vi "Cursor Control.vi"(7 "플랫폼 조합키":T1, 8 "참조":refnum<vi>, 9 "Num Pad":bool, 10 "ScanCode":i16, 11 "error in":errorcluster caption="error out") -> (0 "참조 출력":refnum<vi>, 3 "error out":errorcluster)   [LabVIEW 2020]
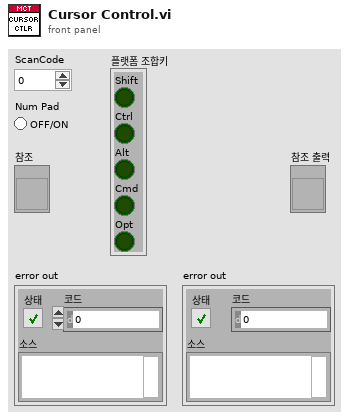
[diagram p1: front panel]
types:
  T1 = cluster{"Shift":bool, "Ctrl":bool, "Alt":bool, "Cmd":bool, "Opt":bool}
  T2 = typedef "LVRowAndColumnTypeDef.ctl" = cluster{"Row":i32, "Column":i32}
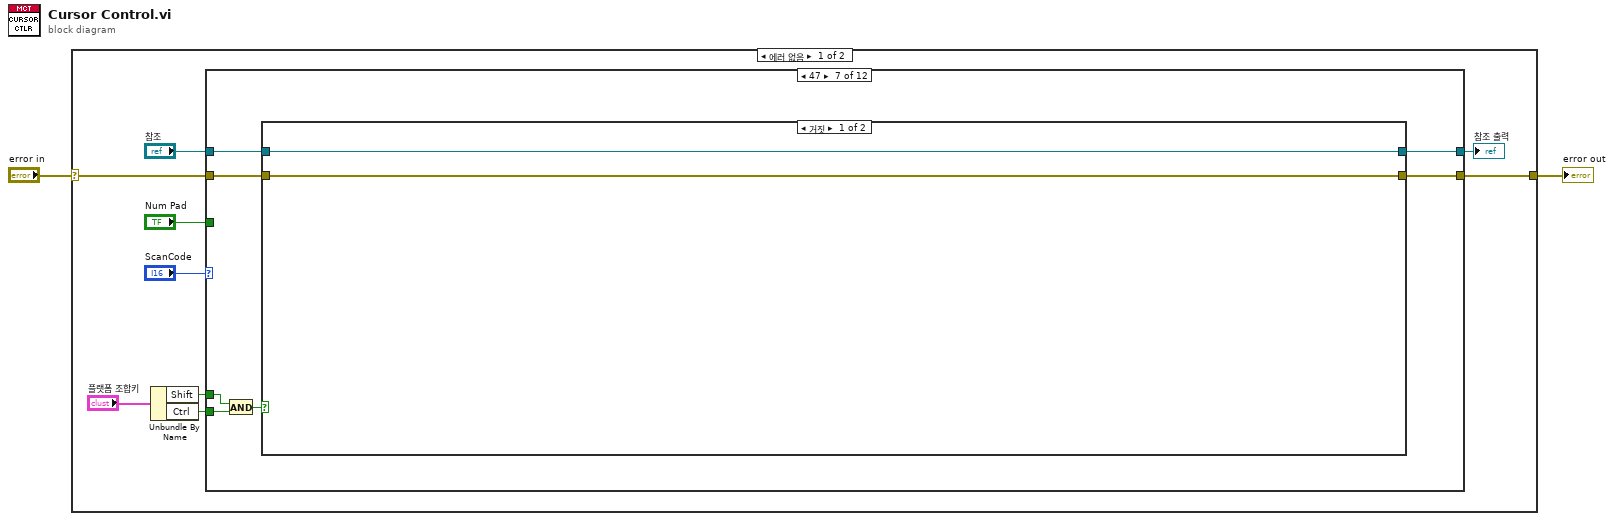
[diagram p0: block diagram]
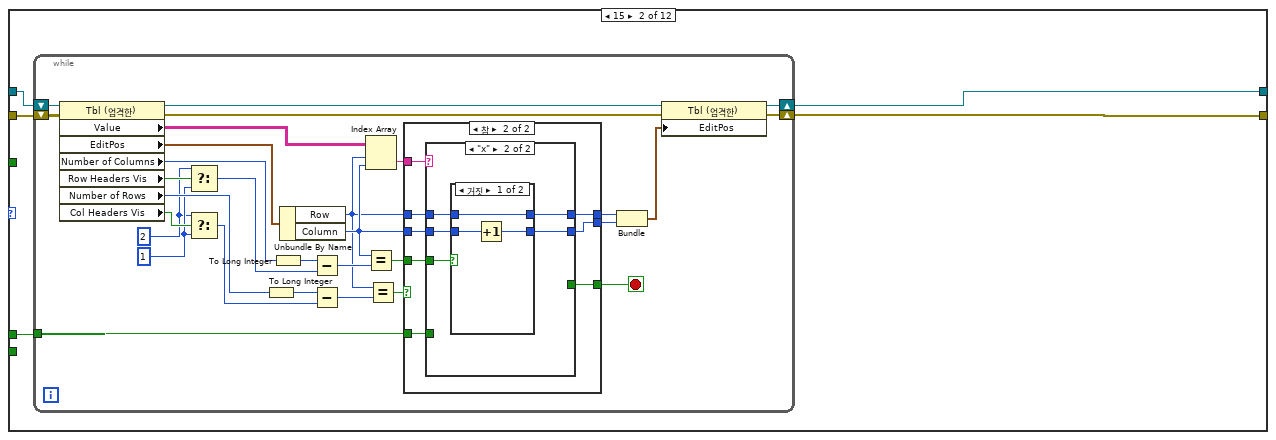
[diagram p3: hidden frame]
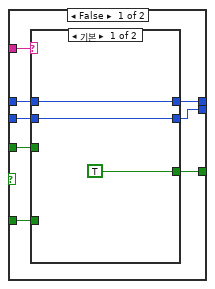
[diagram p4: hidden frame]
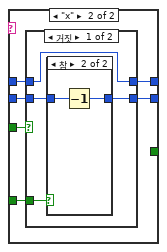
[diagram p5: hidden frame]
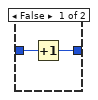
[diagram p6: hidden frame]
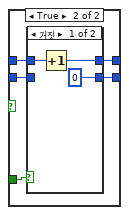
[diagram p7: hidden frame]
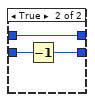
[diagram p8: hidden frame]
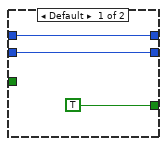
[diagram p9: hidden frame]
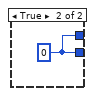
[diagram p10: hidden frame]
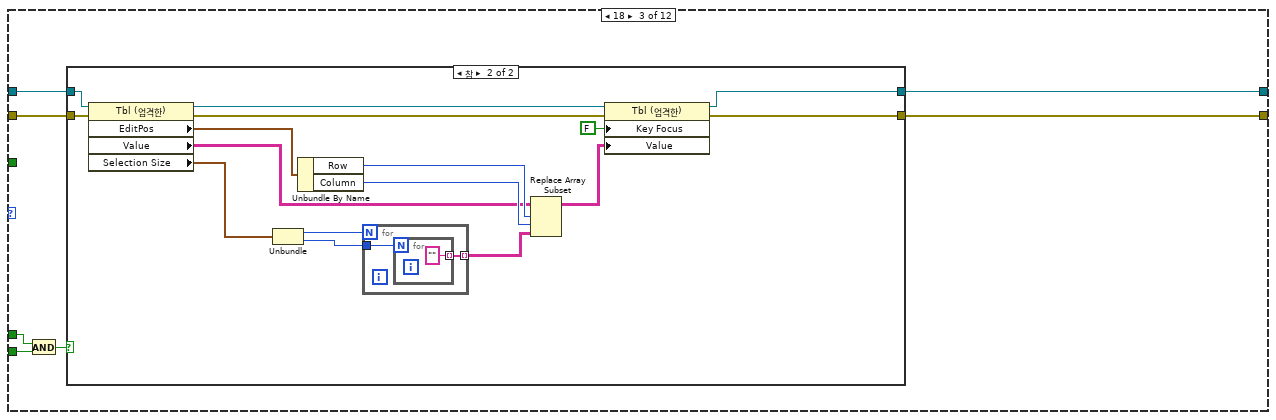
[diagram p11: hidden frame]
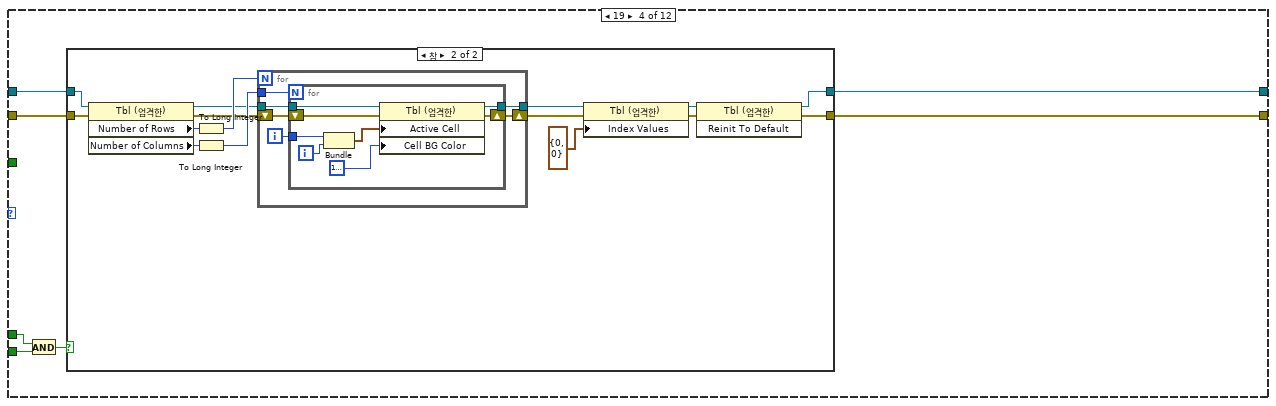
[diagram p13: hidden frame]
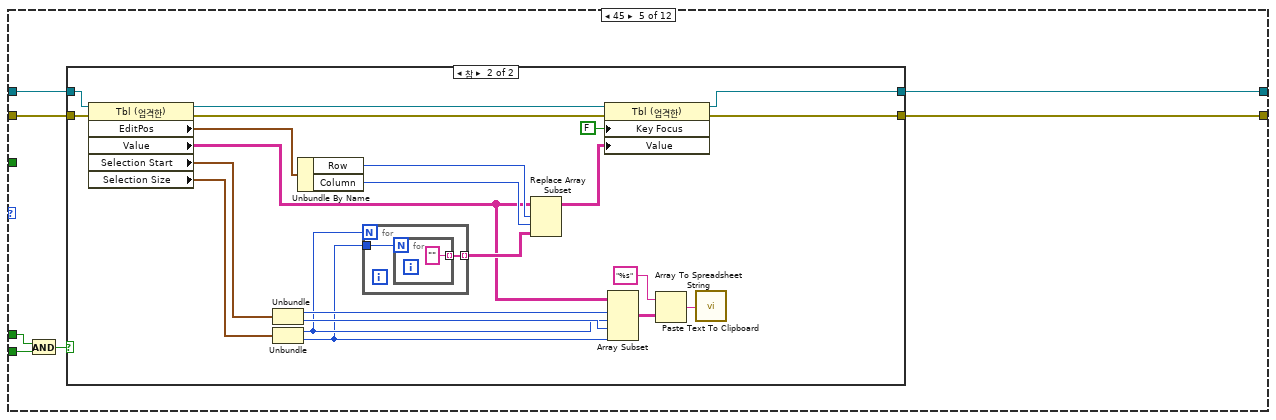
[diagram p15: hidden frame]
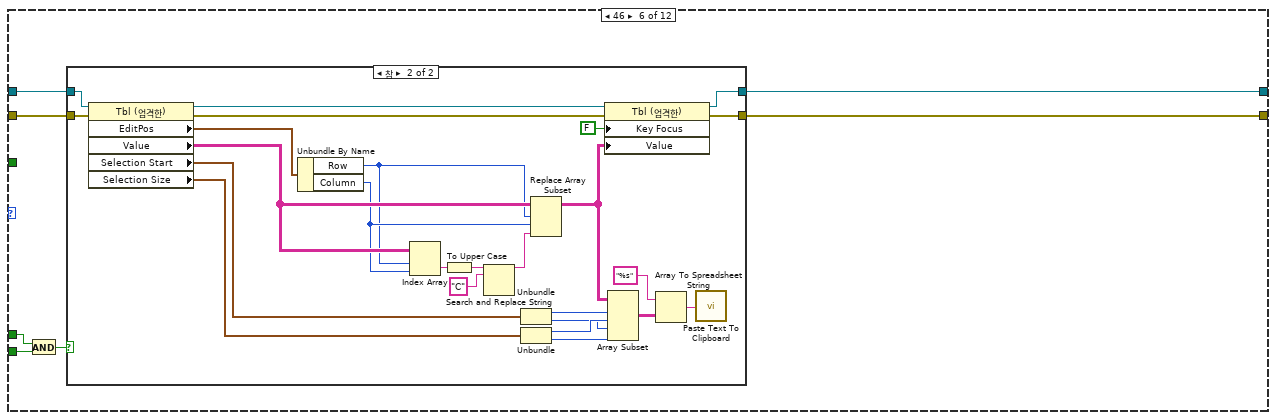
[diagram p17: hidden frame]
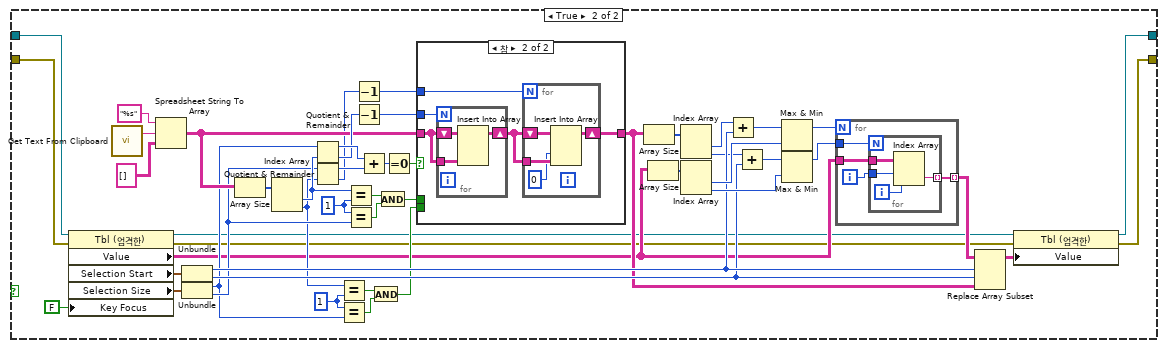
[diagram p19: hidden frame]
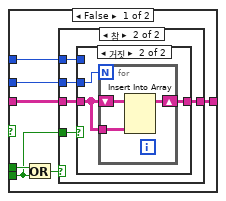
[diagram p20: hidden frame]
diagram:
  n1 = case shown="에러 없음" "error in" {
    selector: "error in" -> [w6 w515]
    tunnel: [w11 w515] -> w2
    frame No Error {
      n2 = Unbundle By Name("플랫폼 조합키") -> ("Shift"=w4:bool, "Ctrl"=w3:bool)
      n3 = case shown="47" "ScanCode" {
        tunnel: w6 -> [w13 w18 w108 w136 w174 w208 w242 w347 w365 w383 w412 w494]
        tunnel: [w13 w16 w106 w134 w172 w206 w240 w346 w364 w382 w411 w493] -> w11
        tunnel: "Num Pad" -> [_ _ _ _ _ _ _ w345 w363 w381 w410 w492]
        tunnel: "참조" -> [w12 w17 w107 w135 w173 w207 w241 w343 w362 w380 w409 w491]
        tunnel: [w12 w15 w105 w133 w171 w205 w239 w344 w361 w379 w408 w490] -> w8
        tunnel: w4 -> [_ w14 w110 w138 w176 w210 w244 _ _ _ w407 _]
        tunnel: w3 -> [_ _ w109 w137 w175 w209 w243 _ _ _ _ _]
        frame Default {
        }
        frame 15 {
          n4 = while {
            shift-right: [w43] -> w16
            shift-left: w18 -> [w47]
            shift-right: [w41] -> w15
            shift-left: w17 -> [w46]
            tunnel: w14 -> [w25]
            stop <- w37 stop-if-true
            w21 = 2 ("y")
            w22 = 1 ("y")
            n5 = property class="Tbl (엄격한)"(reference=w46, error in=w47) -> (reference out=w42:refnum<vi>, error out=w43:errorcluster, "Value"=w45:string[][], "EditPos"=w36:T2, "Number of Columns"=w35:u32, "Row Headers Vis"=w24:bool, "Number of Rows"=w30:u32, "Col Headers Vis"=w23:bool)
            n6 = Select(t=w21, s=w24, f=w22) -> (s? t:f=w20:i32)
            n7 = Select(t=w21, s=w23, f=w22) -> (s? t:f=w19:i32)
            n8 = To Long Integer(number=w30) -> (32bit integer=w26:i32)
            n9 = To Long Integer(number=w35) -> (32bit integer=w28:i32)
            n10 = Unbundle By Name(w36) -> ("Row"=w31:i32, "Column"=w34:i32)
            n11 = Subtract(x=w28, y=w20) -> (x-y=w33:i32)
            n12 = Subtract(x=w26, y=w19) -> (x-y=w29:i32)
            n13 = Index Array(array=w45, index (row)=w31, index (col)=w34) -> (element=w44:string)
            n14 = Equal?(x=w34, y=w33) -> (x = y?=w32:bool)
            n15 = Equal?(x=w31, y=w29) -> (x = y?=w27:bool)
            n16 = case shown="참" w27 {
              tunnel: w44 -> [w55 w91]
              tunnel: [w54 w88] -> w40
              tunnel: [w53 w87] -> w39
              tunnel: [w52 w86] -> w37
              tunnel: w34 -> [w51 w89]
              tunnel: w32 -> [w50 w85]
              tunnel: w31 -> [w49 w90]
              tunnel: w25 -> [w48 w84]
              frame False {
                n17 = case shown="기본" w55 {
                  tunnel: w49 -> [w58 w61]
                  tunnel: w51 -> [w57 w64]
                  tunnel: [w58 w60] -> w54
                  tunnel: [w57 w63] -> w53
                  tunnel: [TRUE _] -> w52
                  tunnel: w50 -> [_ w62]
                  tunnel: w48 -> [_ w59]
                  frame Default {
                  }
                  frame "ⅹ" {
                    n18 = case shown="거짓" w62 {
                      tunnel: w64 -> [w68 w73]
                      tunnel: [w67 w74] -> w63
                      tunnel: w61 -> [w66 w77]
                      tunnel: [w66 w76] -> w60
                      tunnel: w59 -> [w65 w75]
                      frame False {
                        n19 = case shown="참" w65 {
                          tunnel: w68 -> [w70 w72]
                          tunnel: [w69 w71] -> w67
                          frame False {
                            n20 = Increment(x=w70) -> (x+1=w69:i32)
                          }
                          frame True {
                            n21 = Decrement(x=w72) -> (x-1=w71:i32)
                          }
                        }
                      }
                      frame True {
                        n22 = case shown="거짓" w75 {
                          tunnel: w77 -> [w80 w83]
                          tunnel: [w79 w83] -> w76
                          tunnel: [0 w81] -> w74
                          tunnel: w73 -> [_ w82]
                          frame False {
                            n23 = Increment(x=w80) -> (x+1=w79:i32)
                          }
                          frame True {
                            n24 = Decrement(x=w82) -> (x-1=w81:i32)
                          }
                        }
                      }
                    }
                  }
                }
              }
              frame True {
                n25 = case shown="\"ⅹ\"" w91 {
                  tunnel: w90 -> [w94 w96]
                  tunnel: w89 -> [w93 w99]
                  tunnel: [w94 w95] -> w88
                  tunnel: [w93 w98] -> w87
                  tunnel: [TRUE _] -> w86
                  tunnel: w85 -> [_ w97]
                  tunnel: w84 -> [_ _]
                  frame Default {
                  }
                  frame "ⅹ" {
                    n26 = case shown="거짓" w97 {
                      tunnel: w99 -> [w102 _]
                      tunnel: [w101 w103] -> w98
                      tunnel: w96 -> [w100 _]
                      tunnel: [w100 w103] -> w95
                      frame False {
                        n27 = Increment(x=w102) -> (x+1=w101:i32)
                      }
                      frame True {
                        w103 = 0
                      }
                    }
                  }
                }
              }
            }
            n28 = Bundle("Row"=w40, "Column"=w39) -> (w38:cluster{"Row":i32, "Column":i32})  [unwired: 1 in]
            n29 = property class="Tbl (엄격한)"(reference=w42, error in=w43, "EditPos"=w38) -> (reference out=w41:refnum<vi>)  [unwired: 1 out]
          }
        }
        frame 18 {
          n30 = And(x=w110, y=w109) -> (x .and. y?=w104:bool)
          n31 = case shown="참" w104 {
            tunnel: w108 -> [w112 w125]
            tunnel: w107 -> [w111 w126]
            tunnel: [w112 w127] -> w106
            tunnel: [w111 w128] -> w105
            frame False {
            }
            frame True {
              n32 = property class="Tbl (엄격한)"(reference=w126, error in=w125) -> (reference out=w120:refnum<vi>, error out=w121:errorcluster, "EditPos"=w122:T2, "Value"=w113:string[][], "Selection Size"=w117:T2)
              n33 = Unbundle(w117) -> ("Row"=w116:i32, "Column"=w115:i32)
              n34 = Unbundle By Name(w122) -> ("Row"=w123:i32, "Column"=w124:i32)
              n35 = for {
                N: w116 -> [_]
                tunnel: w115 -> [w130]
                tunnel: [w129] -> w114 mode=indexing
                n36 = for {
                  N: w130 -> [_]
                  tunnel: [""] -> w129 mode=indexing
                }
              }
              n37 = Replace Array Subset(array=w113, new element=w114, index (row)=w123, index (col)=w124) -> (w118:string[][])
              n38 = property on="프로퍼티 노드" class="Tbl (엄격한)"(reference=w120, error in=w121, "Key Focus"=FALSE ("키 포커스"), "Value"=w118) -> (reference out=w128:refnum<vi>, error out=w127:errorcluster)
            }
          }
        }
        frame 19 {
          n39 = And(x=w138, y=w137) -> (x .and. y?=w132:bool)
          n40 = case shown="참" w132 {
            tunnel: w136 -> [w140 w149]
            tunnel: w135 -> [w139 w150]
            tunnel: [w140 w141] -> w134
            tunnel: [w139 w142] -> w133
            frame False {
            }
            frame True {
              n41 = property class="Tbl (엄격한)"(reference=w150, error in=w149) -> (reference out=w145:refnum<vi>, error out=w146:errorcluster, "Number of Rows"=w148:u32, "Number of Columns"=w147:u32)
              n42 = To Long Integer(number=w148) -> (32bit integer=w151:i32)
              n43 = To Long Integer(number=w147) -> (32bit integer=w152:i32)
              n44 = for {
                N: w151 -> [_]
                tunnel: w145 -> [w160]
                shift-right: [w159] -> w153
                shift-left: w146 -> [w161]
                tunnel: w152 -> [w157]
                tunnel: [w156] -> w154
                i -> [w158]
                n45 = for {
                  N: w157 -> [_]
                  tunnel: w160 -> [w168]
                  shift-right: [w167] -> w159
                  shift-left: w161 -> [w169]
                  tunnel: w158 -> [w165]
                  tunnel: [w162] -> w156
                  i -> [w164]
                  n46 = Bundle(w165, w164) -> (w166:cluster{i32, i32})  [unwired: 1 in]
                  n47 = property class="Tbl (엄격한)"(reference=w168, error in=w169, "Active Cell"=w166, "Cell BG Color"=u32 16777226) -> (reference out=w162:refnum<vi>, error out=w167:errorcluster)
                }
              }
              n48 = property class="Tbl (엄격한)"(reference=w154, error in=w153, "Index Values"=cluster{i32, i32} {0, 0}) -> (reference out=w144:refnum<vi>, error out=w143:errorcluster)
              n49 = invoke class="Tbl (엄격한)" method="Reinit To Default"(reference=w144, error in=w143) -> (reference out=w142:refnum<vi>, error out=w141:errorcluster)  [unwired: 1 in, 1 out]
            }
          }
        }
        frame 45 {
          n50 = And(x=w176, y=w175) -> (x .and. y?=w170:bool)
          n51 = case shown="참" w170 {
            tunnel: w174 -> [w178 w197]
            tunnel: w173 -> [w177 w198]
            tunnel: [w178 w199] -> w172
            tunnel: [w177 w200] -> w171
            frame False {
            }
            frame True {
              n52 = property class="Tbl (엄격한)"(reference=w198, error in=w197) -> (reference out=w186:refnum<vi>, error out=w187:errorcluster, "EditPos"=w188:T2, "Value"=w179:string[][], "Selection Start"=w191:T2, "Selection Size"=w183:T2)
              n53 = Unbundle(w191) -> ("Row"=w192:i32, "Column"=w193:i32)
              n54 = Unbundle(w183) -> ("Row"=w182:i32, "Column"=w181:i32)
              n55 = Unbundle By Name(w188) -> ("Row"=w189:i32, "Column"=w190:i32)
              n56 = for {
                N: w182 -> [_]
                tunnel: w181 -> [w202]
                tunnel: [w201] -> w180 mode=indexing
                n57 = for {
                  N: w202 -> [_]
                  tunnel: [""] -> w201 mode=indexing
                }
              }
              n58 = Replace Array Subset(array=w179, new element=w180, index (row)=w189, index (col)=w190) -> (w184:string[][])
              n59 = property on="프로퍼티 노드" class="Tbl (엄격한)"(reference=w186, error in=w187, "Key Focus"=FALSE ("키 포커스"), "Value"=w184) -> (reference out=w200:refnum<vi>, error out=w199:errorcluster)
              n60 = Array Subset(array=w179, index (row)=w192, length (row)=w182, index (col)=w193, length (col)=w181) -> (w194:string[][])
              n61 = Array To Spreadsheet String(array=w194, 3:"%s" ("format string")) -> (spreadsheet string=w196:string)  [unwired: 1 in]
              n62 = call "Paste Text To Clipboard.vi"("Text to copy to clipboard"=w196) -> ()  [unwired: 1 out]
            }
          }
        }
        frame 46 {
          n63 = And(x=w210, y=w209) -> (x .and. y?=w204:bool)
          n64 = case shown="참" w204 {
            tunnel: w208 -> [w212 w234]
            tunnel: w207 -> [w211 w235]
            tunnel: [w212 w236] -> w206
            tunnel: [w211 w237] -> w205
            frame False {
            }
            frame True {
              n65 = property class="Tbl (엄격한)"(reference=w235, error in=w234) -> (reference out=w215:refnum<vi>, error out=w216:errorcluster, "EditPos"=w217:T2, "Value"=w233:string[][], "Selection Start"=w225:T2, "Selection Size"=w224:T2)
              n66 = Unbundle By Name(w217) -> ("Row"=w218:i32, "Column"=w220:i32)
              n67 = Index Array(array=w233, index (row)=w218, index (col)=w220) -> (element=w223:string)
              n68 = To Upper Case(1:w223) -> (0:w222:string)
              n69 = Search and Replace String(input string=w222, search string="C" ("검색 문자열")) -> (result string=w219:string)  [unwired: 6 in, 3 out]
              n70 = Unbundle(w225) -> ("Row"=w226:i32, "Column"=w227:i32)
              n71 = Unbundle(w224) -> ("Row"=w232:i32, "Column"=w228:i32)
              n72 = Replace Array Subset(array=w233, new element=w219, index (row)=w218, index (col)=w220) -> (w214:string[][])
              n73 = property on="프로퍼티 노드" class="Tbl (엄격한)"(reference=w215, error in=w216, "Key Focus"=FALSE ("키 포커스"), "Value"=w214) -> (reference out=w237:refnum<vi>, error out=w236:errorcluster)
              n74 = Array Subset(array=w214, index (row)=w226, length (row)=w232, index (col)=w227, length (col)=w228) -> (w229:string[][])
              n75 = Array To Spreadsheet String(array=w229, 3:"%s" ("format string")) -> (spreadsheet string=w231:string)  [unwired: 1 in]
              n76 = call "Paste Text To Clipboard.vi"("Text to copy to clipboard"=w231) -> ()  [unwired: 1 out]
            }
          }
        }
        frame 47 {
          n77 = And(x=w244, y=w243) -> (x .and. y?=w238:bool)
          n78 = case shown="거짓" w238 {
            tunnel: w242 -> [w246 w254]
            tunnel: w241 -> [w245 w253]
            tunnel: [w246 w256] -> w240
            tunnel: [w245 w255] -> w239
            frame False {
            }
            frame True {
              w260 = 1 ("y")
              w268 = 1 ("y")
              n79 = property class="Tbl (엄격한)"(reference=w253, error in=w254, "Key Focus"=FALSE ("키 포커스")) -> (reference out=w247:refnum<vi>, error out=w248:errorcluster, "Value"=w252:string[][], "Selection Start"=w251:T2, "Selection Size"=w250:T2)
              n80 = call "Get Text From Clipboard.vi"() -> ("Text From Clipboard"=w295:string)  [unwired: 1 out]
              n81 = Spreadsheet String To Array(format string="%s", spreadsheet string=w295, array type (2D Dbl)=string[][] []) -> (array=w280:string[][])  [unwired: 1 in]
              n82 = Unbundle(w251) -> ("Row"=w286:i32, "Column"=w285:i32)
              n83 = Unbundle(w250) -> ("Row"=w258:i32, "Column"=w264:i32)
              n84 = Array Size(array=w280) -> (size(s)=w293:i32[])
              n85 = Index Array(array=w293) -> (element #1=w265:i32, element #2=w259:i32)  [unwired: 2 in]
              n86 = Quotient & Remainder(x=w258, y=w265) -> (x-y*floor(x/y)=w284:i32, floor(x/y)=w281:i32)
              n87 = Quotient & Remainder(x=w264, y=w259) -> (x-y*floor(x/y)=w283:i32, floor(x/y)=w273:i32)
              n88 = Equal?(x=w259, y=w260) -> (x = y?=w261:bool)
              n89 = Equal?(x=w260, y=w258) -> (x = y?=w262:bool)
              n90 = Equal?(x=w265, y=w268) -> (x = y?=w267:bool)
              n91 = Equal?(x=w268, y=w264) -> (x = y?=w266:bool)
              n92 = Decrement(x=w273) -> (x-1=w272:i32)
              n93 = Decrement(x=w281) -> (x-1=w274:i32)
              n94 = Add(x=w284, y=w283) -> (x+y=w282:i32)
              n95 = And(x=w261, y=w262) -> (x .and. y?=w257:bool)
              n96 = And(x=w267, y=w266) -> (x .and. y?=w263:bool)
              n97 = Equal To 0?(x=w282) -> (x = 0?=w279:bool)
              n98 = case shown="참" w279 {
                tunnel: w274 -> [w309 w335]
                tunnel: w280 -> [w311 w334]
                tunnel: [w308 w333] -> w277
                tunnel: w272 -> [w310 w331]
                tunnel: w263 -> [w307 _]
                tunnel: w257 -> [w306 _]
                frame False {
                  n99 = Or(x=w307, y=w306) -> (x .or. y?=w305:bool)
                  n100 = case shown="참" w305 {
                    tunnel: w311 -> [w312 w317]
                    tunnel: w306 -> [_ w316]
                    tunnel: w310 -> [_ w315]
                    tunnel: w309 -> [_ w314]
                    tunnel: [w312 w313] -> w308
                    frame False {
                    }
                    frame True {
                      n101 = case shown="거짓" w316 {
                        tunnel: w317 -> [w320 w327]
                        tunnel: w315 -> [w319 _]
                        tunnel: w314 -> [_ w325]
                        tunnel: [w318 w326] -> w313
                        frame True {
                          n102 = for {
                            N: w319 -> [_]
                            shift-right: [w323] -> w318
                            shift-left: w320 -> [w324]
                            tunnel: w320 -> [w322]
                            n103 = Insert Into Array(array=w324, index (col)=0 ("비활성화된 인덱스 (열)"), new element=w322) -> (w323:string[][])  [unwired: 1 in]
                          }
                        }
                        frame False {
                          n104 = for {
                            N: w325 -> [_]
                            shift-right: [w329] -> w326
                            shift-left: w327 -> [w330]
                            tunnel: w327 -> [w328]
                            n105 = Insert Into Array(array=w330, new element=w328) -> (w329:string[][])  [unwired: 2 in]
                          }
                        }
                      }
                    }
                  }
                }
                frame True {
                  n106 = for {
                    N: w335 -> [_]
                    shift-right: [w340] -> w332
                    shift-left: w334 -> [w342]
                    tunnel: w334 -> [w341]
                    n107 = Insert Into Array(array=w342, new element=w341) -> (w340:string[][])  [unwired: 2 in]
                  }
                  n108 = for {
                    N: w331 -> [_]
                    shift-right: [w337] -> w333
                    shift-left: w332 -> [w339]
                    tunnel: w332 -> [w338]
                    n109 = Insert Into Array(array=w339, index (col)=0 ("비활성화된 인덱스 (열)"), new element=w338) -> (w337:string[][])  [unwired: 1 in]
                  }
                }
              }
              n110 = Array Size(array=w277) -> (size(s)=w278:i32[])
              n111 = Array Size(array=w252) -> (size(s)=w292:i32[])
              n112 = Index Array(array=w278) -> (element #1=w276:i32, element #2=w275:i32)  [unwired: 2 in]
              n113 = Index Array(array=w292) -> (element #1=w288:i32, element #2=w287:i32)  [unwired: 2 in]
              n114 = Add(x=w276, y=w286) -> (x+y=w290:i32)
              n115 = Add(x=w275, y=w285) -> (x+y=w289:i32)
              n116 = Max & Min(x=w290, y=w288) -> (max(x,y)=w271:i32)  [unwired: 1 out]
              n117 = Max & Min(x=w289, y=w287) -> (max(x,y)=w270:i32)  [unwired: 1 out]
              n118 = for {
                N: w271 -> [_]
                tunnel: [w300] -> w269 mode=indexing
                tunnel: w270 -> [w298]
                tunnel: w252 -> [w297]
                i -> [w299]
                n119 = for {
                  N: w298 -> [_]
                  tunnel: [w302] -> w300 mode=indexing
                  tunnel: w299 -> [w304]
                  tunnel: w297 -> [w301]
                  i -> [w303]
                  n120 = Index Array(array=w301, index (row)=w304, index (col)=w303) -> (element=w302:string)
                }
              }
              n121 = Replace Array Subset(array=w269, new element=w277, index (row)=w286, index (col)=w285) -> (w291:string[][])
              n122 = property class="Tbl (엄격한)"(reference=w247, error in=w248, "Value"=w291) -> (reference out=w255:refnum<vi>, error out=w256:errorcluster)
            }
          }
        }
        frame 72 {
          n123 = case shown="거짓" w345 {
            tunnel: w347 -> [w358 w360]
            tunnel: [w356 w360] -> w346
            tunnel: [w350 w359] -> w344
            tunnel: w343 -> [w348 w359]
            frame False {
              n124 = property on="프로퍼티 노드" class="Tbl (엄격한)"(reference=w348, error in=w358) -> (reference out=w349:refnum<vi>, error out=w357:errorcluster, "EditPos"=w354:T2)
              n125 = Unbundle By Name(w354) -> ("Row"=w353:i32, "Column"=w351:i32)
              n126 = Decrement(x=w353) -> (x-1=w352:i32)
              n127 = Bundle By Name(cluster=w354, "Row"=w352, "Column"=w351) -> (w355:T2)
              n128 = property on="프로퍼티 노드" class="Tbl (엄격한)"(reference=w349, error in=w357, "EditPos"=w355) -> (reference out=w350:refnum<vi>, error out=w356:errorcluster)
            }
            frame True {
            }
          }
        }
        frame 75 {
          n129 = case shown="거짓" w363 {
            tunnel: w365 -> [w376 w378]
            tunnel: [w374 w378] -> w364
            tunnel: w362 -> [w368 w377]
            tunnel: [w366 w377] -> w361
            frame False {
              n130 = property on="프로퍼티 노드" class="Tbl (엄격한)"(reference=w368, error in=w376) -> (reference out=w367:refnum<vi>, error out=w375:errorcluster, "EditPos"=w372:T2)
              n131 = Unbundle By Name(w372) -> ("Row"=w370:i32, "Column"=w371:i32)
              n132 = Decrement(x=w371) -> (x-1=w369:i32)
              n133 = Bundle By Name(cluster=w372, "Row"=w370, "Column"=w369) -> (w373:T2)
              n134 = property on="프로퍼티 노드" class="Tbl (엄격한)"(reference=w367, error in=w375, "EditPos"=w373) -> (reference out=w366:refnum<vi>, error out=w374:errorcluster)
            }
            frame True {
            }
          }
        }
        frame 77 {
          n135 = case shown="거짓" w381 {
            tunnel: w383 -> [w401 w406]
            tunnel: [w399 w406] -> w382
            tunnel: w380 -> [w392 w405]
            tunnel: [w390 w405] -> w379
            frame False {
              n136 = property on="프로퍼티 노드" class="Tbl (엄격한)"(reference=w392, error in=w401) -> (reference out=w391:refnum<vi>, error out=w400:errorcluster, "EditPos"=w397:T2, "Number of Columns"=w389:u32, "Row Headers Vis"=w387:bool)
              n137 = Select(t=u32 2, s=w387, f=u32 1 ("y")) -> (s? t:f=w385:u32)
              n138 = Unbundle By Name(w397) -> ("Row"=w396:i32, "Column"=w393:i32)
              n139 = Subtract(x=w389, y=w385) -> (x-y=w388:u32)
              n140 = Equal?(x=w393, y=w388) -> (x = y?=w394:bool)
              n141 = case shown="참" w394 {
                tunnel: w393 -> [w403 w404]
                tunnel: [w402 w404] -> w395
                frame False {
                  n142 = Increment(x=w403) -> (x+1=w402:i32)
                }
                frame True {
                }
              }
              n143 = Bundle By Name(cluster=w397, "Row"=w396, "Column"=w395) -> (w398:T2)
              n144 = property on="프로퍼티 노드" class="Tbl (엄격한)"(reference=w391, error in=w400, "EditPos"=w398) -> (reference out=w390:refnum<vi>, error out=w399:errorcluster)
            }
            frame True {
            }
          }
        }
        frame 78 {
          # "+"
          n145 = case shown="참" w410 {
            tunnel: w412 -> [w414 w452]
            tunnel: [w414 w442] -> w411
            tunnel: w409 -> [w413 w448]
            tunnel: [w413 w443] -> w408
            tunnel: w407 -> [_ w423]
            frame False {
            }
            frame True {
              w427 = 1 ("y")
              w428 = 2 ("y")
              n146 = property on="프로퍼티 노드" class="Tbl (엄격한)"(reference=w448, error in=w452) -> (reference out=w447:refnum<vi>, error out=w451:errorcluster, "EditPos"=w449:T2, "Number of Rows"=w446:u32, "Col Headers Vis"=w431:bool, "Number of Columns"=w432:u32, "Row Headers Vis"=w429:bool, "Value"=w437:string[][])
              n147 = Select(t=w428, s=w431, f=w427) -> (s? t:f=w430:i32)
              n148 = Select(t=w428, s=w429, f=w427) -> (s? t:f=w425:i32)
              n149 = To Long Integer(number=w446) -> (32bit integer=w424:i32)
              n150 = To Long Integer(number=w432) -> (32bit integer=w426:i32)
              n151 = Unbundle By Name(w449) -> ("Row"=w420:i32, "Column"=w417:i32)
              n152 = Subtract(x=w424, y=w430) -> (x-y=w416:i32)
              n153 = Subtract(x=w426, y=w425) -> (x-y=w415:i32)
              n154 = Equal?(x=w416, y=w420) -> (x = y?=w422:bool)
              n155 = Equal?(x=w415, y=w417) -> (x = y?=w421:bool)
              n156 = case shown="참" w423 {
                tunnel: w422 -> [w458 _]
                tunnel: w421 -> [w457 _]
                tunnel: w420 -> [w456 w472]
                tunnel: [w455 w475] -> w419
                tunnel: [w454 w474] -> w418
                tunnel: w417 -> [w453 w473]
                tunnel: w416 -> [_ w471]
                tunnel: w415 -> [_ w470]
                frame False {
                  n157 = case shown="거짓" w458 {
                    tunnel: w457 -> [w462 _]
                    tunnel: w456 -> [_ w468]
                    tunnel: [w461 w469] -> w455
                    tunnel: [w460 w467] -> w454
                    tunnel: w453 -> [w459 w467]
                    frame True {
                      n158 = case shown="참" w462 {
                        tunnel: [0 w466] -> w461
                        tunnel: [w463 w466] -> w460
                        tunnel: w459 -> [w464 _]
                        frame False {
                          n159 = Increment(x=w464) -> (x+1=w463:i32)
                        }
                        frame True {
                          w466 = 0
                        }
                      }
                    }
                    frame False {
                      n160 = Increment(x=w468) -> (x+1=w469:i32)
                    }
                  }
                }
                frame True {
                  n161 = case shown="0" w472 {
                    selector: w472 -> [w478 w481]
                    tunnel: [w476 w484] -> w475
                    tunnel: [w477 w483] -> w474
                    tunnel: w473 -> [w477 w482]
                    tunnel: w471 -> [_ w480]
                    tunnel: w470 -> [_ w479]
                    frame Default {
                      n162 = Decrement(x=w478) -> (x-1=w476:i32)
                    }
                    frame 0 {
                      n163 = case shown="기본" w482 {
                        selector: w482 -> [w486 _]
                        tunnel: [w485 w489] -> w484
                        tunnel: [w487 w488] -> w483
                        tunnel: w481 -> [_ _]
                        tunnel: w480 -> [w485 w489]
                        tunnel: w479 -> [_ w488]
                        frame Default {
                          n164 = Decrement(x=w486) -> (x-1=w487:i32)
                        }
                        frame 0 {
                        }
                      }
                    }
                  }
                }
              }
              n165 = Index Array(array=w437, index (row)=w420, index (col)=w417) -> (element=w435:string)
              n166 = Bundle By Name(cluster=w449, "Row"=w419, "Column"=w418) -> (w450:T2)
              n167 = property on="프로퍼티 노드" class="Tbl (엄격한)"(reference=w447, error in=w451, "EditPos"=w450) -> (reference out=w444:refnum<vi>, error out=w445:errorcluster, "Value"=w439:string[][])
              n168 = Index Array(array=w439, index (row)=w420, index (col)=w417) -> (element=w441:string)
              n169 = Search and Replace String(input string=w441, search string="+" ("검색 문자열")) -> (result string=w434:string)  [unwired: 6 in, 3 out]
              n170 = Empty String/Path?(string/path=w434) -> (empty?=w436:bool)
              n171 = Select(t=w435, s=w436, f=w434) -> (s? t:f=w433:string)
              n172 = Replace Array Subset(array=w439, new element=w433, index (row)=w420, index (col)=w417) -> (w438:string[][])
              n173 = property on="프로퍼티 노드" class="Tbl (엄격한)"(reference=w444, error in=w445, "Value"=w438) -> (reference out=w443:refnum<vi>, error out=w442:errorcluster)
            }
          }
        }
        frame 80 {
          n174 = case shown="거짓" w492 {
            tunnel: w494 -> [w509 w514]
            tunnel: [w507 w514] -> w493
            tunnel: w491 -> [w500 w513]
            tunnel: [w498 w513] -> w490
            frame False {
              n175 = property on="프로퍼티 노드" class="Tbl (엄격한)"(reference=w500, error in=w509) -> (reference out=w499:refnum<vi>, error out=w508:errorcluster, "EditPos"=w505:T2, "Number of Rows"=w497:u32)
              n176 = Unbundle By Name(w505) -> ("Row"=w502:i32, "Column"=w504:i32)
              n177 = Subtract(x=w497, y=u32 2) -> (x-y=w496:u32)
              n178 = Equal?(x=w502, y=w496) -> (x = y?=w501:bool)
              n179 = case shown="거짓" w501 {
                tunnel: w502 -> [w511 w512]
                tunnel: [w510 w512] -> w503
                frame False {
                  n180 = Increment(x=w511) -> (x+1=w510:i32)
                }
                frame True {
                }
              }
              n181 = Bundle By Name(cluster=w505, "Row"=w503, "Column"=w504) -> (w506:T2)
              n182 = property on="프로퍼티 노드" class="Tbl (엄격한)"(reference=w499, error in=w508, "EditPos"=w506) -> (reference out=w498:refnum<vi>, error out=w507:errorcluster)
            }
            frame True {
            }
          }
        }
      }
      "참조 출력" <- w8
    }
    frame Error {
    }
  }
  "error out" <- w2
